vi "Write PAR_index.vi"(9 "Reg":string, 10 "EnumsPAR":string[](array[string]), 11 "bronkhorst_reg in":refnum<class "bronkhorst_reg_2.lvclass">) -> (2 "Find":bool, 3 "bronkhorst_reg out":refnum<class "bronkhorst_reg_2.lvclass">)   [LabVIEW 2019, in "control.lvlib" / "bronkhorst_reg_2.lvclass"]
uses:
  bronkhorst_reg_2.lvclass
  bronkhorst_reg_2.lvclass/bronkhorst_reg_2.ctl
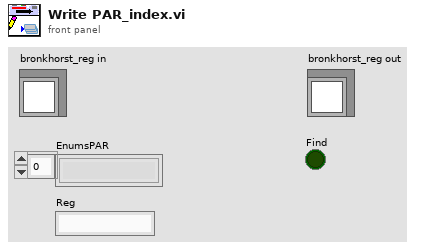
[diagram p1: front panel]
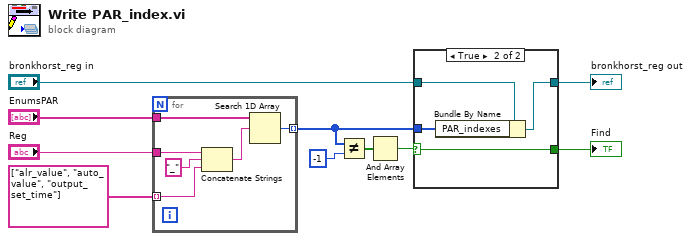
[diagram p0: block diagram]
diagram:
  n1 = for {
    tunnel: "EnumsPAR" -> [w16]
    tunnel: "Reg" -> [w15]
    tunnel: [w13] -> w1 mode=indexing
    tunnel: string[] ["alr_value", "auto_value", "output_set_time"] -> [w11] mode=indexing
    n2 = Concatenate Strings(w15, "_" ("string"), w11) -> (w14:string)
    n3 = Search 1D Array(1D array=w16, element=w14) -> (index of element=w13:i32)  [unwired: 1 in]
  }
  n4 = Not Equal?(x=w1, y=-1 ("index of element")) -> (x != y?=w8:bool[])
  n5 = And Array Elements(Boolean array=w8) -> (logical AND=w2:bool)
  n6 = case shown="True" w2 {
    selector: w2 -> [w17 w20]
    tunnel: "bronkhorst_reg in" -> [w18 w22]
    tunnel: [w18 w21] -> w5
    tunnel: [w17 w20] -> w7
    tunnel: w1 -> [_ w19]
    frame False {
    }
    frame True {
      n7 = Bundle By Name(cluster=w22, "PAR_indexes"=w19) -> (w21:refnum<class "bronkhorst_reg_2.lvclass">)
    }
  }
  "bronkhorst_reg out" <- w5
  "Find" <- w7
